vi "Preselection_KBC21_31.vi"(0 "SI804.lvclass in":refnum<class "SI804.lvclass">, 2 "3 JSB30 DG801\nXA11":bool, 3 "3 JSB30 DG802\nXA11":bool, 5 "error in":errorcluster) -> (14 "SI804.lvclass out":refnum<class "SI804.lvclass">, 16 "PreSelec KBC21":bool, 17 "PreSelec KBC31":bool, 19 "error out":errorcluster)   [LabVIEW 2022 SP3, in "SI804.lvclass"]
uses:
  SI804.lvclass
  SI804.lvclass/SI804.ctl
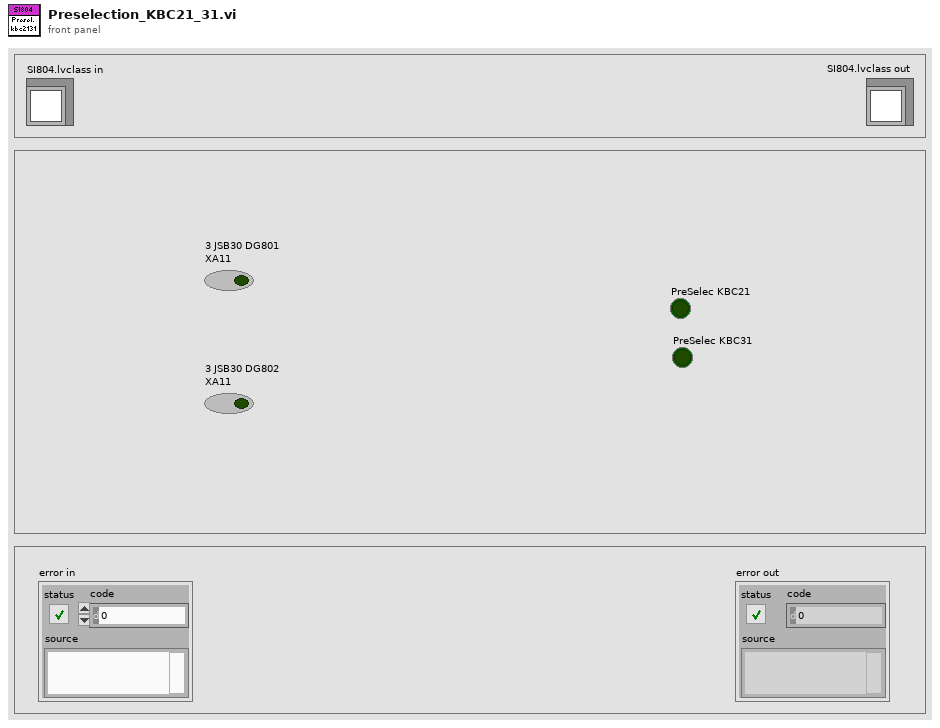
[diagram p1: front panel]
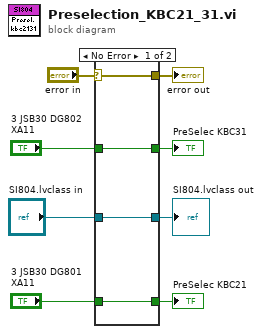
[diagram p0: block diagram]
diagram:
  n1 = case shown="No Error" "error in" {
    selector: "error in" -> [w10 w14]
    tunnel: "3 JSB30 DG801\nXA11" -> [w12 _]
    tunnel: "3 JSB30 DG802\nXA11" -> [w11 _]
    tunnel: [w12 _] -> w4
    tunnel: [w11 _] -> w3
    tunnel: [w10 w14] -> w5
    tunnel: "SI804.lvclass in" -> [w9 w13]
    tunnel: [w9 w13] -> w1
    frame No Error {
    }
    frame Error {
    }
  }
  "error out" <- w5
  "PreSelec KBC21" <- w4
  "PreSelec KBC31" <- w3
  "SI804.lvclass out" <- w1
